vi "Option2_with_case_in_loop.vi"() -> ()   [LabVIEW 2022 SP3]
doc: "This example performs writes and reads on a serial port, as directed by the user. You can press the Write and Read buttons, and change the Read Count, while the example is running.\n\nThe parameters set for the serial port must match the parameters of the connected instrument or device. In this example, the Read Count parameter specifies the number of bytes that the serial port reads. If there were more bytes at the port than the specified number, those bytes would not be read. If there were less bytes at the port than the specified number, you would receive a timeout error.\n\nThis example expands upon the flow control options for XON and XOFF, allowing the user to choose those control characters. Also, the user can enable or disable a termination character. Some devices require a termination character in order to identify the end of command strings. Some devices send a termination character to signify the end of data to be read. This example shows how you can end the Read operation once a termination character is detected in the buffer and/or append a termination character at the end of the Write data."
uses:
  PolyStat_LabVIEW_control_project/Command_buttons.ctl
  Applications/National Instruments/LabVIEW 2022 64-bit/examples/Instrument IO/Serial/support/Serial - Settings.ctl
  Applications/National Instruments/LabVIEW 2022 64-bit/examples/Instrument IO/Serial/support/Serial - XON-XOFF Characters.ctl
  Applications/National Instruments/LabVIEW 2022 64-bit/examples/Instrument IO/Serial/support/Serial - ASCII Characters.ctl
  <vilib>/Instr/_visa.llb/VISA Configure Serial Port (Instr).vi
panel:
  in  "Stop":bool
  in  "Temperature\nto set":dbl
  in  "Command Radio\nButtons":T1
  out "Response":string
  in  "Write":bool
  in  "Read":bool
  in  "VISA resource name":refnum<visa-resource-name>="COM1"
  # "------------------------\nPROGRAM EXECUTION   \n------------------------\n1. Connect PolyStat controller to PC via RS232 cable and choose corresponding port in 'VISA resource name'\n2. Set the time to poll which decides the time interval between each write-read pair or how often the command must be written and read\n3. Choose command to run by clicking the Radio buttons (can be changed during run). Refer the COMMANDS description for correct usage.\n4. Set the read and write buttons to ON for continuous polling mode\n5. Response can be observed on the given Response indicator\n6. Saved log PolyState_LabVIEW_log.txt can be found at LabVIEW default directory\n\nNOTE:\n> Only one command can be sent at a time\n> Program execution stops if controller response is negative\n> Program execution stops with error if no response is received from controller within 12 seconds after write\n> Time to poll cannot be changed during run, it is only read once at start"
  # "--------------\nCOMMANDS\n--------------\nP0 => Power off and standby\nP1 => Power on from standby\nF? => query fluid temperature\nS? => query current set temperature\nSn => set temperature to value n (change number between -40 to 105)\nValue of n should be given in 'Temperature to set' control\nUC => set unit to Celsius\nUF => set unit to Fahrenheit"
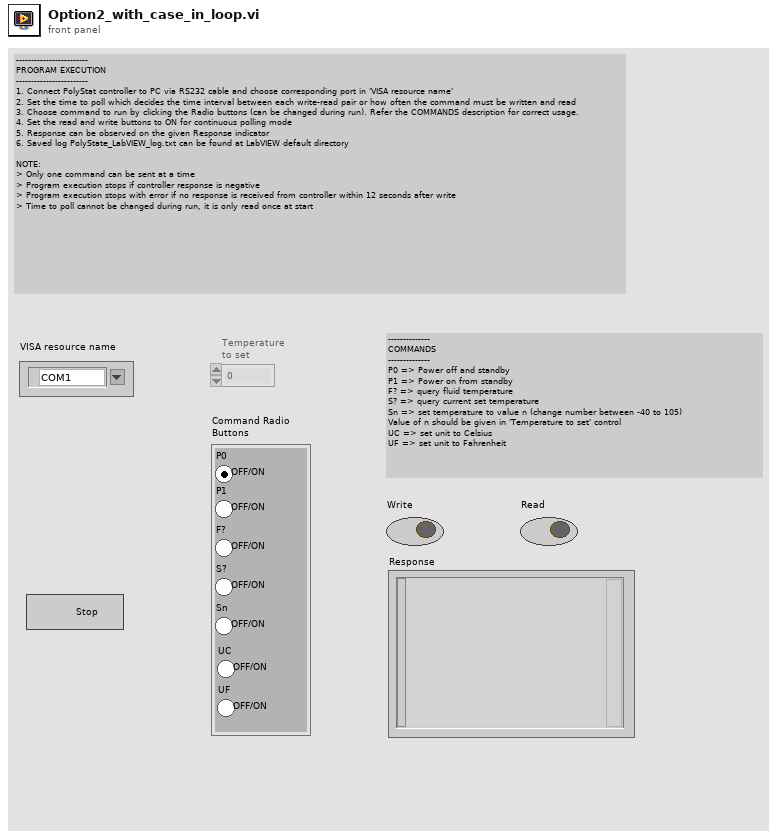
[diagram p1: front panel]
types:
  T1 = typedef "Command_buttons.ctl" = enum32{"P0", "P1", "F?", "S?", "Sn", "UC", "UF"}
  T2 = enum16{"open", "replace", "create", "open or create", "replace or create", "replace or create with confirmation"}
  T3 = typedef "Serial - XON-XOFF Characters.ctl" = cluster{"XON":T4, "XOFF":T4}
  T4 = typedef "Serial - ASCII Characters.ctl" = enum16{"NUL", "SOH", "STX", "ETX", "EOT", "ENQ", "ACK", "BEL", "BS", "HT", "LF", "VT", "FF", "CR", "SO", "SI", "DLE", "DC1", "DC2", "DC3", "DC4", "NAK", "SYN", "ETB", "CAN", "EM", "SUB", "ESC", "FS", "GS", "RS", "US", "SP", "!", "\"", "#", "$", "%", "&", "'", "(", ")", "*", "+", ",", "- (-)", ".", "/", "0", "1", "2", "3", "4", "5", "6", "7", "8", "9", ":", ";", "<", "=", ">", "?", "@", "A", "B", "C", "D", "E", "F", "G", "H", "I", "J", "K", "L", "M", "N", "O", "P", "Q", "R", "S", "T", "U", "V", "W", "X", "Y", "Z", "[", "\\", "]", "^", "_", "`", "a", "b", "c", "d", "e", "f", "g", "h", "i", "j", "k", "l", "m", "n", "o", "p", "q", "r", "s", "t", "u", "v", "w", "x", "y", "z", "{", "|", "}", "~"}
  T5 = typedef "Serial - Settings.ctl" = cluster{"baud rate":u32, "data bits":u16, "parity":enum16{"None", "Odd", "Even", "Mark", "Space"}, "stop bits":u16, "flow control":u16}
  T6 = enum8{"Enabled", "Disabled", "Disabled and Grayed Out"}
  T7 = typedef "Written_command.ctl" = string
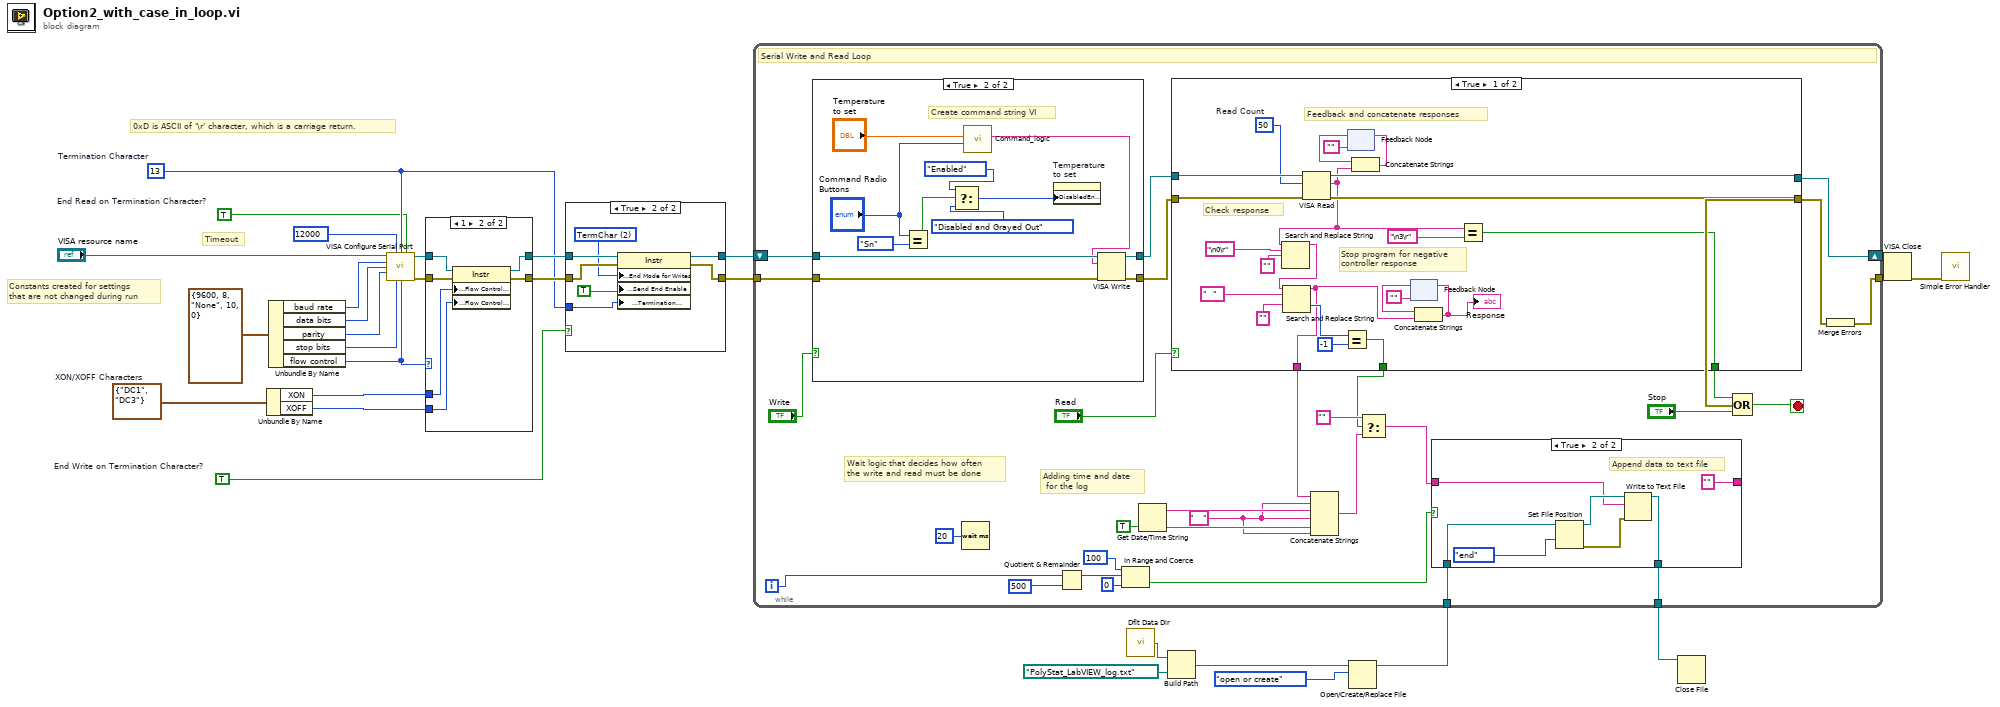
[diagram p0: block diagram]
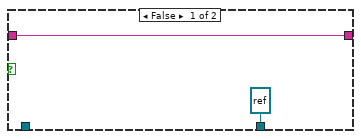
[diagram p4: hidden frame]
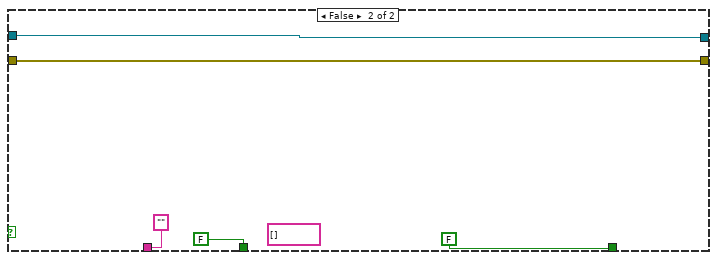
[diagram p6: hidden frame]
diagram:
  w8 = T3 {"XON"=enum."DC1", "XOFF"=enum."DC3"}  # XON/XOFF Characters
  w9 = TRUE  # End Write on Termination Character?
  w10 = TRUE  # End Read on Termination Character?
  w11 = u8 13  # Termination Character
  # "Constants created for settings\nthat are not changed during run"
  # "Timeout"
  # "0xD is ASCII of '\\r' character, which is a carriage return."
  n1 = Unbundle By Name(w8) -> ("XON"=w18:T4, "XOFF"=w17:T4)
  n2 = Unbundle By Name(T5 {"baud rate"=9600, "data bits"=8, "parity"=enum."None", "stop bits"=10, "flow control"=0} ("input cluster")) -> ("baud rate"=w23:u32, "data bits"=w24:u16, "parity"=w25:enum16{"None", "Odd", "Even", "Mark", "Space"}, "stop bits"=w26:u16, "flow control"=w19:u16)
  n3 = call-poly "VISA Configure Serial Port"("VISA resource name"="VISA resource name", "timeout (10sec)"=u32 12000, "termination char\n(0xA = '\\n' = LF)"=w11, "Enable Termination\nChar (T)"=w10, "baud rate (9600)"=w23, "data bits (8)"=w24, "parity (0:none)"=w25, "stop bits (10: 1 bit)"=w26, "flow control (0:none)"=w19) -> ("VISA resource name out"=w27:refnum<visa-resource-name>, "error out"=w28:errorcluster)  [unwired: 1 in, 4 out]
  n4 = case shown="1" w19 {
    tunnel: [w30 w37] -> w16
    tunnel: [w31 w36] -> w14
    tunnel: w28 -> [w30 w35]
    tunnel: w27 -> [w31 w34]
    tunnel: w18 -> [_ w33]
    tunnel: w17 -> [_ w32]
    frame Default {
    }
    frame 1 {
      n5 = property class="Instr"(reference=w34, error in=w35, "Serial Settings:Flow Control XON Character"=w33, "Serial Settings:Flow Control XOFF Character"=w32) -> (reference out=w36:refnum<visa-resource-name>, error out=w37:errorcluster)
    }
  }
  n6 = case shown="True" w9 {
    tunnel: w14 -> [w38 w46]
    tunnel: w16 -> [w39 w45]
    tunnel: [w38 w44] -> w13
    tunnel: [w39 w43] -> w15
    tunnel: w11 -> [_ w41]
    frame False {
    }
    frame True {
      w42 = u16 2 items=["None", "LastBit", "TermChar", "Break"] ("Serial Settings:Serial End Mode for Writes")
      n7 = property class="Instr"(reference=w46, error in=w45, "Serial Settings:End Mode for Writes"=w42, "Message Based Settings:Send End Enable"=TRUE, "Message Based Settings:Termination Character"=w41) -> (reference out=w44:refnum<visa-resource-name>, error out=w43:errorcluster)
    }
  }
  n8 = call <vilib>:"Dflt Data Dir.vi"() -> ("App:Default Data Directory"=w6:path)
  n9 = Build Path(base path=w6, name or relative path=path "PolyStat_LabVIEW_log.txt" ("default name")) -> (appended path=w3:path)
  n10 = Open/Create/Replace File(file path (use dialog)=w3, operation (0:open)=T2."open or create") -> (refnum out=w2:refnum<file>)  [unwired: 4 in, 2 out]
  n11 = while {
    shift-right: [w76] -> w20
    shift-left: w13 -> [w75]
    tunnel: w15 -> [w74]
    tunnel: [w65] -> w21
    tunnel: w2 -> [w55]
    tunnel: [w54] -> w1
    i -> [w52]
    stop <- w69 stop-if-true
    w59 = "   " ("string")
    # "Adding time and date\n for the log"
    # "Wait logic that decides how often\nthe write and read must be done"
    # "Serial Write and Read Loop"
    n12 = case shown="True" "Write" {
      tunnel: w75 -> [w87 w99]
      tunnel: w74 -> [w86 w98]
      tunnel: [w87 w97] -> w68
      tunnel: [w86 w96] -> w73
      frame False {
      }
      frame True {
        # "Create command string VI"
        n13 = Equal?(x="Command Radio\nButtons", y=Command_buttons."Sn") -> (x = y?=w89:bool)
        n14 = Select(t=T6."Enabled" ("Disabled"), s=w89, f=T6."Disabled and Grayed Out" ("Disabled")) -> (s? t:f=w88:T6)
        n15 = call "Command_logic.vi"("Command Radio Buttons"="Command Radio\nButtons", "Temperature\nto set"="Temperature\nto set") -> ("Written command"=w94:T7)  [unwired: 9 in]
        n16 = property on="Temperature\nto set" class="DigNum (strict)"("DisabledEnum"=w88) -> ()  [unwired: 2 in, 2 out]
        n17 = VISA Write(VISA resource name=w99, write buffer=w94, error in (no error)=w98) -> (VISA resource name out=w97:refnum<visa-resource-name>, error out=w96:errorcluster)  [unwired: 1 out]
      }
    }
    n18 = Wait (ms)(milliseconds to wait=u32 20) -> ()  [unwired: 1 out]
    n19 = Quotient & Remainder(x=w52, y=500) -> (x-y*floor(x/y)=w51:i32)  [unwired: 1 out]
    n20 = In Range and Coerce(upper limit=100, x=w51, lower limit=0) -> (In Range?=w50:bool)  [unwired: 1 out]
    n21 = Get Date/Time String(want seconds? (F)=TRUE) -> (date string=w61:string, time string=w60:string)  [unwired: 2 in]
    n22 = case shown="True" "Read" {
      tunnel: [w120 w127] -> w76
      tunnel: w68 -> [w122 w127]
      tunnel: [w119 w126] -> w66
      tunnel: w73 -> [w121 w126]
      tunnel: [w101 ""] -> w58
      tunnel: [w114 FALSE] -> w70
      tunnel: [w100 FALSE] -> w63
      frame True {
        w116 = u32 50  # Read Count
        # "Check response"
        # "Feedback and concatenate responses"
        # "Stop program for negative\ncontroller response"
        n23 = VISA Read(VISA resource name=w122, byte count=w116, error in (no error)=w121) -> (VISA resource name out=w120:refnum<visa-resource-name>, read buffer=w111:string, error out=w119:errorcluster)  [unwired: 1 out]
        n24 = Search and Replace String(input string=w111, search string="\n0\r" ("regular expression (\"\")"), replace string="" ("replace string (\"\")")) -> (result string=w107:string)  [unwired: 5 in, 3 out]
        n25 = Search and Replace String(input string=w107, search string="  " ("regular expression (\"\")"), replace string="" ("replace string (\"\")")) -> (result string=w101:string, offset past replacement=w106:i32)  [unwired: 5 in, 2 out]
        n26 = Equal?(x=w106, y=-1) -> (x = y?=w100:bool)
        n27 = feedback #1("") -> (w118:string)
        n28 = Concatenate Strings(w118, w111) -> (w110:string)
        n29 = feedback-in #1(w110) -> ()
        n30 = feedback #2("") -> (w103:string)
        n31 = Concatenate Strings(w103, w101) -> (w104:string)
        "Response" <- w104
        n32 = feedback-in #2(w104) -> ()
        n33 = Equal?(x=w111, y="\n3\r" ("regular expression (\"\")")) -> (x = y?=w114:bool)
      }
      frame False {
        (unwired) string[] []
      }
    }
    n34 = Concatenate Strings(w58, w59, w61, w59, w60, w59) -> (w57:string)
    n35 = Select(t="", s=w63, f=w57) -> (s? t:f=w49:string)
    n36 = case shown="True" w50 {
      tunnel: w55 -> [_ w82]
      tunnel: [refnum<file> refnum ("refnum out") w81] -> w54
      tunnel: w49 -> [w78 w80]
      tunnel: [w78 "" ("t")] -> _
      frame False {
      }
      frame True {
        # "Append data to text file"
        n37 = Set File Position(refnum=w82, from (0:start)=enum16{"start", "end", "current"}."end") -> (refnum out=w84:refnum<file>, error out=w85:errorcluster)  [unwired: 2 in]
        n38 = Write to Text File(file (use dialog)=w84, text=w80, error in=w85) -> (refnum out=w81:refnum<file>)  [unwired: 1 in, 2 out]
      }
    }
    n39 = Compound Arithmetic op=OR(w70, w66, "Stop") -> (w69:bool)
    n40 = Merge Errors(w66) -> (w65:errorcluster)
  }
  n41 = Close File(refnum=w1) -> ()  [unwired: 1 in, 2 out]
  n42 = VISA Close(VISA resource name=w20, error in (no error)=w21) -> (error out=w22:errorcluster)
  n43 = call <vilib>:"Simple Error Handler.vi"("error in (no error)"=w22) -> ()  [unwired: 1 in, 8 out]
